vi "SecuenceHasBeenSent.vi"(7 "Max ID":i32, 9 "TestName":T1, 10 "IDS":string[](array[string]), 11 "Result Set":string[][](array[string])) -> ()   [LabVIEW 2020, in "Settings.lvlib"]
doc: "_____\nCreated using Delacor QMH Event Scripter 6.0.0.121."
uses:
  Settings.lvlib
  TestName--control.ctl
  SecuenceHasBeenSent Argument--cluster.ctl
panel:
  in  "error in":errorcluster
  out "error out":errorcluster
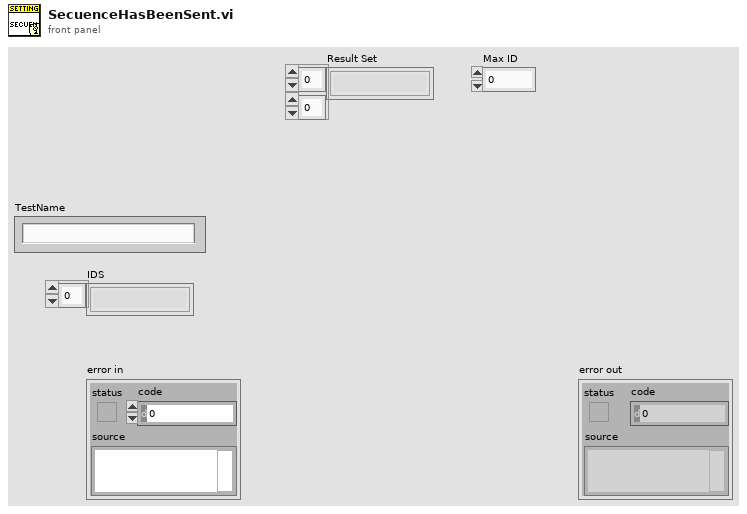
[diagram p1: front panel]
types:
  T1 = typedef "TestName--control.ctl" = string
  T2 = typedef "Settings.lvlib/SecuenceHasBeenSent Argument--cluster.ctl" = cluster{"IDS":string[], "Result Set":string[][], "Max ID":i32, "TestName":T1}
  T3 = typedef "Settings.lvlib/Broadcast Events--cluster.ctl" = cluster{"Module Did Init":refnum<user-event>, "Status Updated":refnum<user-event>, "Error Reported":refnum<user-event>, "Module Did Stop":refnum<user-event>, "Update Module Execution Status":refnum<user-event>, "NameTest":refnum<user-event>, "SecuenceHasBeenSent":refnum<user-event>, "TypeSignal":refnum<user-event>}
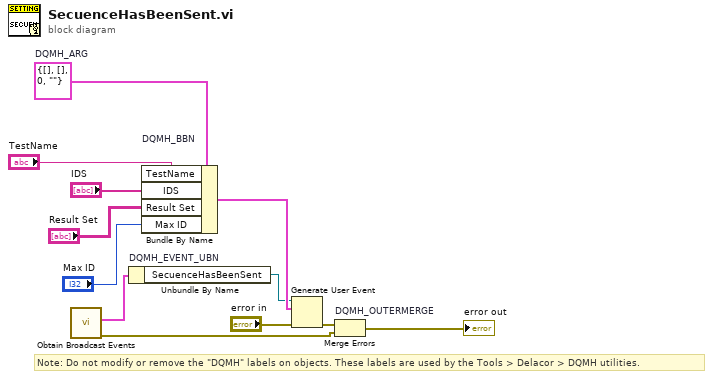
[diagram p0: block diagram]
diagram:
  w7 = T2 {"IDS"=[], "Result Set"=[], "Max ID"=0, "TestName"=""}  # DQMH_ARG
  # "Note: Do not modify or remove the \"DQMH\" labels on objects. These labels are used by the Tools > Delacor > DQMH utilities."
  n1 = call "Obtain Broadcast Events.vi"() -> ("error out"=w3:errorcluster, "Settings Broadcast Events"=w2:T3)  [unwired: 10 in]
  n2 = Unbundle By Name "DQMH_EVENT_UBN"(w2) -> ("SecuenceHasBeenSent"=w9:refnum<user-event>)
  n3 = Bundle By Name "DQMH_BBN"(cluster=w7, "TestName"="TestName", "IDS"="IDS", "Result Set"="Result Set", "Max ID"="Max ID") -> (w10:T2)
  n4 = Generate User Event(user event=w9, event data cluster=w10, error in="error in") -> (error out=w8:errorcluster)  [unwired: 1 in, 1 out]
  n5 = Merge Errors "DQMH_OUTERMERGE"(w8, w3) -> (→"error out":errorcluster)
